vi "Lake Shore Cryotronics 218 Sensor Reading.vi"() -> ()   [LabVIEW 2017]
doc: "This VI was designed to demonstrate typical usage of sub VIs containing the more common 218 functions. The VI first configures the input group and input to be read using the LSCI 218 Config input.vi. Time is then provided for the instrument to configure the input group and input. Finally, the selected input is read."
uses:
  Lake Shore Cryotronics 218.lvlib
panel:
  in  "Input Curve (0:None)":u16(ring) items=["None", "DT-470", "DT-500", "CTI Diode", "Empty Standard Diode", "Empty Standard Diode", "PT-100", "PT-1000", "Empty Standard Platinum", "Empty Standard Platinum", "Unused", "Unused", "Unused", "Unused", "Unused", "Unused", "Unused", "Unused", "Unused", "Unused", "Unused", "User Curve 1", "User Curve 2", "User Curve 3", "User Curve 4", "User Curve 5", "User Curve 6", "User Curve 7", "User Curve 8"]
  in  "Input (1)":dbl=1.0 min=1.0 max=8.0 step=1.0
  in  "Input Type (0:2.5V Diode)":u16(ring) items=["2.5V Diode", "7.5V Diode", "250 Ohm Platinum", "500 Ohm Platinum", "5K Ohm Platinum", "Cernox"]
  in  "Input Group (0:Inputs 1-4)":u16(ring) items=["Inputs 1-4", "Inputs 5-8"]
  out "VISA resource name out":refnum<visa-resource-name>
  out "error out":errorcluster
  in  "error in (no error)":errorcluster
  in  "VISA resource name":refnum<visa-resource-name>
  in  "Data Source (0:Kelvin)":u16(ring) items=["Kelvin", "Celsius", "Sensor Units", "Linear Data"]
  out "Sensor Reading":dbl format="%.4f"
  # "© 2005 National Instruments.  ALL RIGHTS RESERVED."
  # "218 Temperature Monitor"
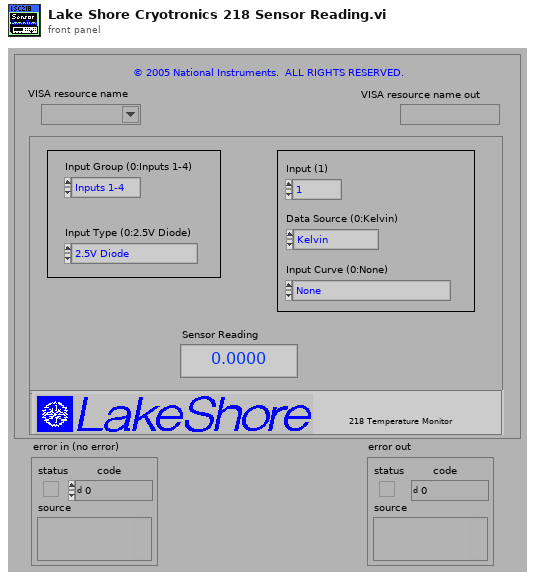
[diagram p1: front panel]
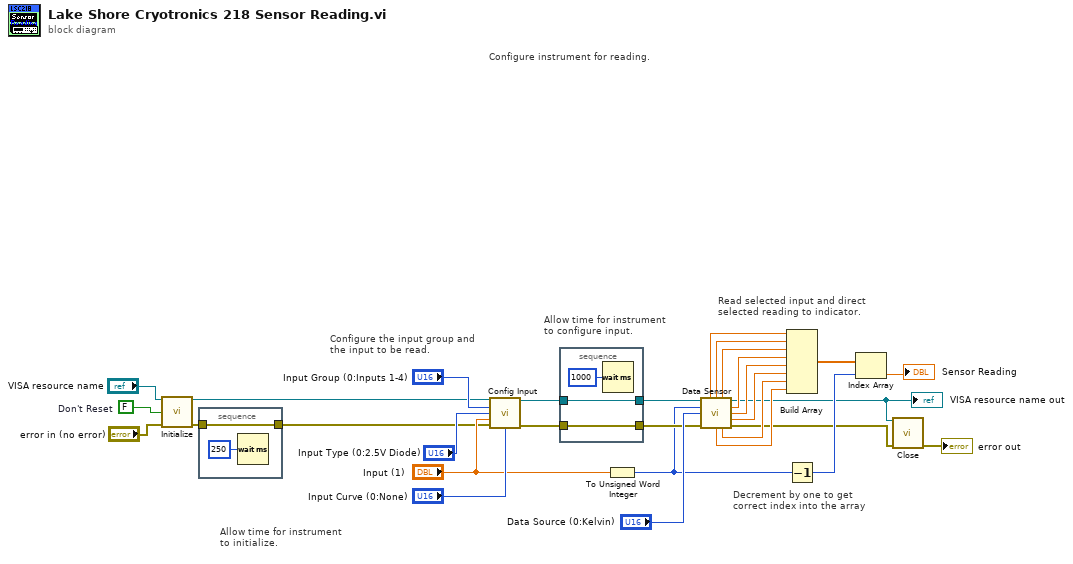
[diagram p0: block diagram]
diagram:
  w6 = FALSE  # Don't Reset
  # "Allow time for instrument \nto initialize."
  # "Decrement by one to get \ncorrect index into the array"
  # "Read selected input and direct\nselected reading to indicator."
  # "Allow time for instrument\nto configure input."
  # "Configure instrument for reading."
  # "Configure the input group and\nthe input to be read."
  n1 = call "Initialize.vi"("VISA resource name"="VISA resource name", "Reset (T: Reset)"=w6, "error in (no error)"="error in (no error)") -> ("VISA resource name out"=w4:refnum<visa-resource-name>, "error out"=w5:errorcluster)  [unwired: 11 in]
  n2 = stacked-sequence {
    tunnel: w5 -> [w31]
    tunnel: [w31] -> w3
    frame #0 {
      n3 = Wait (ms)(milliseconds to wait=u32 250) -> ()  [unwired: 1 out]
    }
  }
  n4 = call "Config Input.vi"("VISA resource name"=w4, "Input Group (0:Inputs 1-4)"="Input Group (0:Inputs 1-4)", "Sensor Type (0:2.5V Diode)"="Input Type (0:2.5V Diode)", "Input (1)"="Input (1)", "error in (no error)"=w3, "Input Curve (0:None)"="Input Curve (0:None)") -> ("VISA resource name out"=w11:refnum<visa-resource-name>, "error out"=w26:errorcluster)  [unwired: 8 in]
  n5 = stacked-sequence {
    tunnel: w26 -> [w35]
    tunnel: [w35] -> w25
    tunnel: w11 -> [w33]
    tunnel: [w33] -> w10
    frame #0 {
      n6 = Wait (ms)(milliseconds to wait=u32 1000) -> ()  [unwired: 1 out]
    }
  }
  n7 = To Unsigned Word Integer(number="Input (1)") -> (unsigned 16bit integer=w22:u16)
  n8 = call "Data Sensor.vi"("VISA resource name"=w10, "Input (0:All)"=w22, "Data Source (0:Kelvin)"="Data Source (0:Kelvin)", "error in (no error)"=w25) -> ("Input 1"=w23:dbl, "Input 2"=w21:dbl, "Input 3"=w20:dbl, "VISA resource name out"=w8:refnum<visa-resource-name>, "Input 4"=w19:dbl, "Input 5"=w18:dbl, "Input 6"=w17:dbl, "Input 8"=w15:dbl, "Input 7"=w16:dbl, "error out"=w9:errorcluster)  [unwired: 2 in]
  "VISA resource name out" <- w8
  n9 = Build Array(w23, w21, w20, w19, w18, w17, w16, w15) -> (w14:dbl[])
  n10 = Decrement(x=w22) -> (x-1=w13:u16)
  n11 = Index Array(array=w14, index=w13) -> (element=→"Sensor Reading":dbl)
  n12 = call "Close.vi"("VISA resource name"=w8, "error in (no error)"=w9) -> ("error out"=→"error out":errorcluster)  [unwired: 13 in]
